vi "get_position.vi"(11 "Range in":refnum<class "Block.lvclass">) -> (2 "position":i32, 3 "Range out":refnum<class "Block.lvclass">)   [LabVIEW 2020, in "variant.lvlib" / "Block.lvclass"]
uses:
  Block.lvclass
  Block.lvclass/Block.ctl
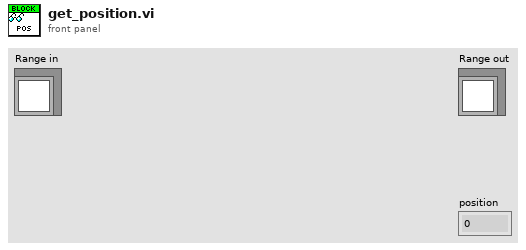
[diagram p1: front panel]
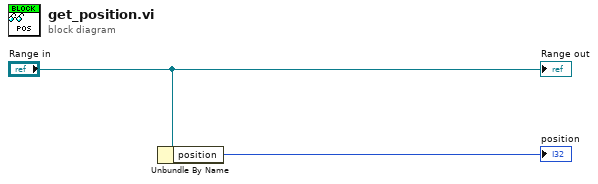
[diagram p0: block diagram]
diagram:
  n1 = Unbundle By Name("Range in") -> ("position"=→"position":i32)
  "Range out" <- "Range in"
